vi "Enquire.vi"(8 "error in (no error)":errorcluster, 11 "Socket.TCP in":refnum<class "Socket.TCP.lvclass">) -> (0 "error out":errorcluster, 3 "Socket.TCP out":refnum<class "Socket.TCP.lvclass">)   [LabVIEW 2014, in "Socket.lvlib" / "Socket.TCP.lvclass"]
doc: "Sends Ascii \"ENQ\" \\0x05 to the receiver.\n\nThis can be used to discover if a connection was shut down unexpectedly. \n\nCaution should be used that the ENQ is recognized by a receiver as Enquire and not as a bit of data or a packet length byte."
uses:
  Socket.TCP.lvclass
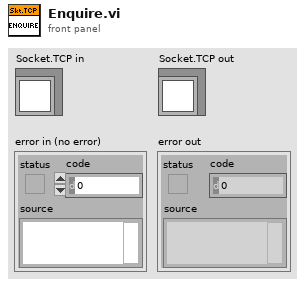
[diagram p1: front panel]
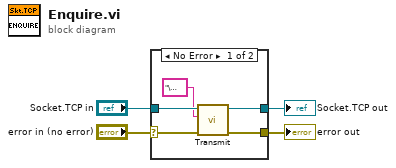
[diagram p0: block diagram]
diagram:
  n1 = case shown="No Error" "error in (no error)" {
    selector: "error in (no error)" -> [w8 w10]
    tunnel: [w8 w10] -> w3
    tunnel: [w5 w9] -> w1
    tunnel: "Socket.TCP in" -> [w7 w9]
    frame No Error {
      n2 = call-dynamic "Transmit.vi"("data"="\u0005" ("Data"), "Socket.TCP in"=w7) -> ("Socket.TCP out"=w5:refnum<class "Socket.TCP.lvclass">)  [unwired: 7 in, 2 out]
    }
    frame Error {
    }
  }
  "error out" <- w3
  "Socket.TCP out" <- w1
